vi "Pre Launch Init.vi"(11 "TcpServer in":refnum<class "TcpServer.lvclass">) -> (0 "error out":errorcluster, 3 "TcpServer out":refnum<class "TcpServer.lvclass">)   [LabVIEW 2022 SP3, in "TcpServer.lvlib" / "TcpServer.lvclass"]
doc: "(<B>Filename</B>: Actor Framework.lvlib:Actor.lvclass:Pre Launch Init.vi)\n\nDefines behavior that occurs after the Launch Actor method is invoked but before the actor's Actor Core method begins running.\n\nThe Pre Launch Init method is guaranteed to finish before the Launch Actor method returns to its caller and before the actor itself receives any messages. Any references that the Pre Launch Init method obtains are guaranteed to have the same lifetime as the actor itself. Any errors that the Pre Launch Init method returns will abort the launch.\n\nBy default, this method does nothing. A descendant class may override it to define behavior."
uses:
  TcpServer.lvclass
  DataReceived/DataReceived.lvclass
  TcpServer.lvclass/TcpServer.ctl
  LoggingActor/Source/LoggingActor/LoggingActor/LoggingActor.lvclass
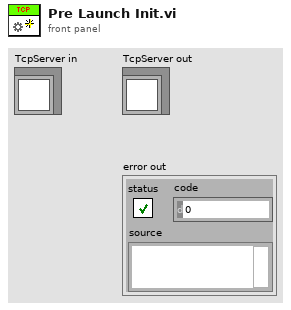
[diagram p1: front panel]
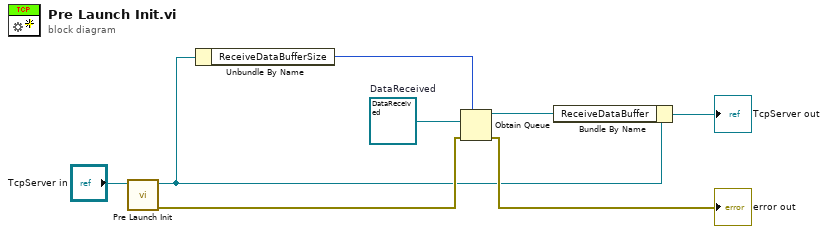
[diagram p0: block diagram]
diagram:
  w4 = refnum<class "DataReceived.lvclass"> refnum  # DataReceived
  n1 = call-parent "Pre Launch Init.vi"("LoggingActor in"="TcpServer in") -> ("error out"=w7:errorcluster, "LoggingActor out"=w2:refnum<class "TcpServer.lvclass">)  [unwired: 9 in]
  n2 = Unbundle By Name(w2) -> ("ReceiveDataBufferSize"=w1:i32)
  n3 = Obtain Queue(max queue size (-1, unlimited)=w1, element data type=w4, error in (no error)=w7) -> (queue out=w5:refnum<queue>, error out=→"error out":errorcluster)  [unwired: 2 in, 1 out]
  n4 = Bundle By Name(cluster=w2, "ReceiveDataBuffer"=w5) -> (→"TcpServer out":refnum<class "TcpServer.lvclass">)
